vi "NotifyIcon Process.vi"(8 "error in (no error)":errorcluster, 10 "ItemTag":string, 11 "Model in":refnum<class "Model.lvclass">) -> (0 "error out":errorcluster, 3 "Model out":refnum<class "Model.lvclass">)   [LabVIEW 2021, in "Model.lvlib" / "Model.lvclass"]
uses:
  Model.lvclass
  Model.lvclass/Model.ctl
  <userlib>/John_Lib/Control/Panel State.ctl
  6fa144c1-b21d-4c7d-8ae2-4db209a0c860.vi
  df4c223b-0860-4833-9d57-1994cce9cdf4.vi
  <userlib>/John_Lib/AMC_FW/Send Local Message.vi
  <userlib>/John_Lib/AMC_FW/Create Single Message.vi
  <userlib>/John_Lib/AMC_FW/Update Message Routing Info.vi
  <userlib>/John_Lib/AMC_FW/String to Array.vi
  <userlib>/John_Lib/AMC_FW/Send Message.vi
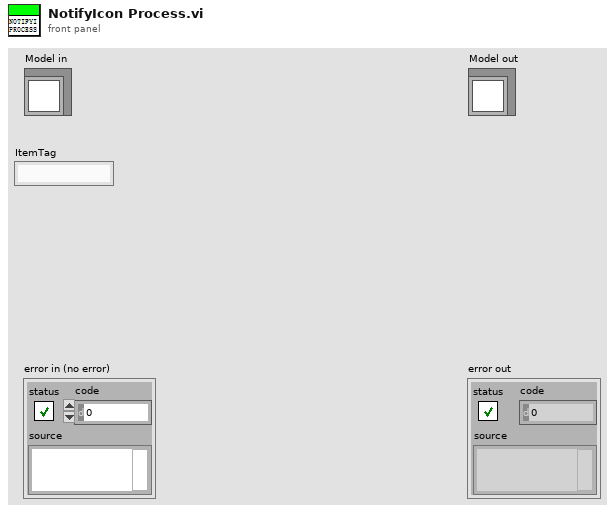
[diagram p1: front panel]
types:
  T1 = typedef "AMC_FW.lvlib/Queue.ctl" = cluster{"Q":T2, "Name":string}
  T2 = typedef "AMC_FW.lvlib/Message Queue.ctl" = refnum<queue>
  T3 = typedef "Panel State.ctl" = string
  T4 = enum32{"Invalid", "Standard", "Closed", "Hidden", "Minimized", "Maximized"}
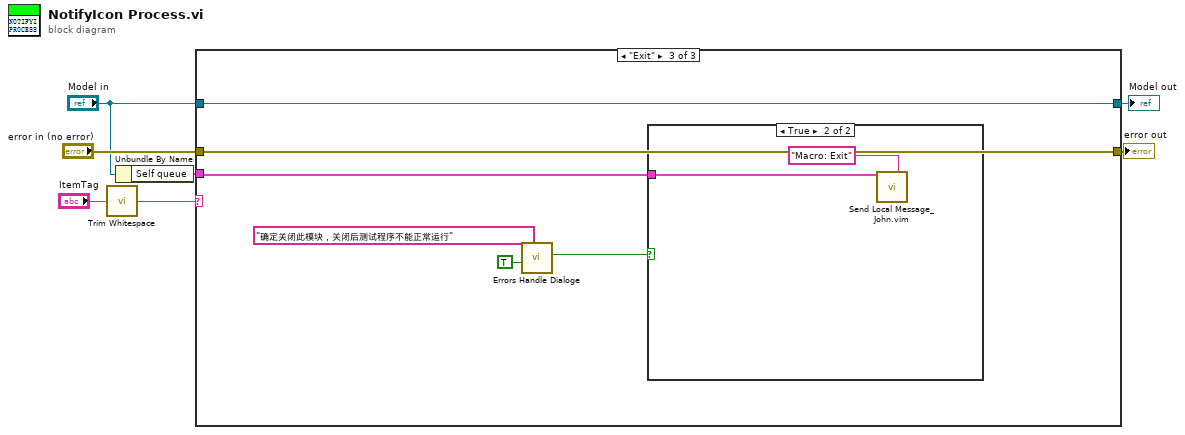
[diagram p0: block diagram]
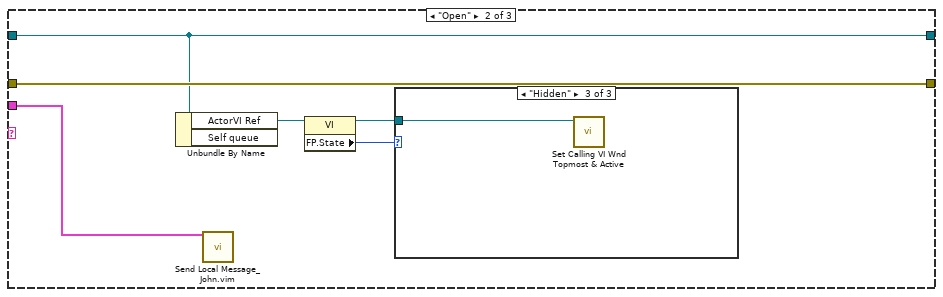
[diagram p3: hidden frame]
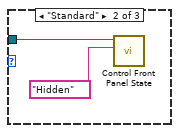
[diagram p5: hidden frame]
diagram:
  n1 = call <vilib>:"Trim Whitespace.vi"("string"="ItemTag") -> ("trimmed string"=w6:string)  [unwired: 1 in]
  n2 = Unbundle By Name("Model in") -> ("Self queue"=w1:T1)
  n3 = case shown="\"Exit\"" w6 {
    tunnel: "Model in" -> [w9 w14 w24]
    tunnel: [w9 w14 w24] -> w5
    tunnel: "error in (no error)" -> [w8 w15 w23]
    tunnel: [w8 w15 w23] -> w3
    tunnel: w1 -> [_ w11 w19]
    frame "False", Default {
    }
    frame "Open" {
      n4 = Unbundle By Name(w14) -> ("ActorVI Ref"=w13:refnum<vi>)  [unwired: 1 out]
      n5 = call "Send Local Message_John.vim"("Queue In"=w11) -> ()  [unwired: 12 in, 3 out]
      n6 = property class="VI"(reference=w13) -> (reference out=w10:refnum<vi>, "FP.State"=w12:T4)  [unwired: 1 in, 1 out]
      n7 = case shown="\"Hidden\"" w12 {
        tunnel: w10 -> [_ w17 w18]
        frame "Invalid", Default {
        }
        frame "Standard" {
          n8 = call <userlib>:"Control Front Panel State.vi"("Argument"=T3 "Hidden", "Core.Current VI Reference"=w17) -> ()  [unwired: 8 in, 2 out]
        }
        frame "Hidden" {
          n9 = call <userlib>:"Set Calling VI Wnd Topmost & Active.vi"("vi reference"=w18) -> ()  [unwired: 10 in, 1 out]
        }
      }
    }
    frame "Exit" {
      n10 = call <userlib>:"Errors Handle Dialoge.vi"("DisplayDialog"=TRUE, "Message"="确定关闭此模块，关闭后测试程序不能正常运行") -> ("OK?"=w20:bool)  [unwired: 8 in, 1 out]
      n11 = case shown="True" w20 {
        tunnel: w19 -> [_ w26]
        frame False {
        }
        frame True {
          n12 = call "Send Local Message_John.vim"("Queue In"=w26, "Elements in Front"="Macro: Exit") -> ()  [unwired: 11 in, 3 out]
        }
      }
    }
  }
  "error out" <- w3
  "Model out" <- w5
